vi "ADCPro_error_global.vi"() -> ()   [LabVIEW 2010, in "ErrorLog.lvlib"]
uses:
  ErrorLog.lvlib
panel:
  in  "Error Description - Custom":string[](array[string])=["Invalid Plugin Directory", "Invalid Plugin Directory", "Invalid Plugin INI File", "Error locating selected plugin"]
  in  "Error Codes - Custom":i32[](array[numeric])=[6010, 6011, 6012, 6019]
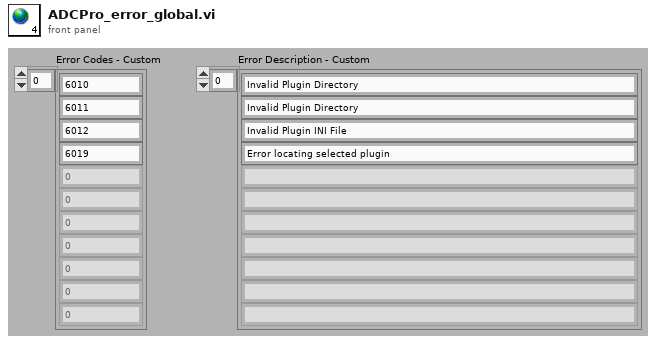
[diagram p1: front panel]
diagram:
